vi "dequetosend.vi"(8 "error in (no error)":errorcluster, 11 "queue":refnum<queue>) -> (0 "error out":errorcluster, 3 "String to be sent":string)   [LabVIEW 2016]
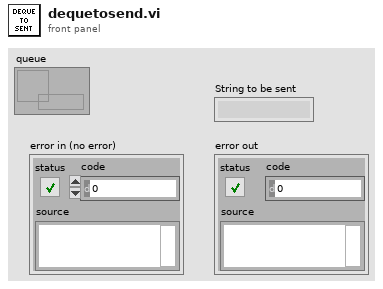
[diagram p1: front panel]
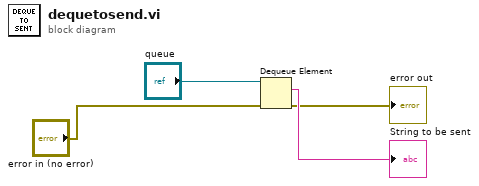
[diagram p0: block diagram]
diagram:
  n1 = Dequeue Element(queue="queue", error in (no error)="error in (no error)") -> (element=→"String to be sent":string, error out=→"error out":errorcluster)  [unwired: 1 in, 2 out]
